vi "NI VeriStand - Close Multiple Waveforms Read Session (CDB).vi"(8 "error in (no error)":errorcluster, 11 "Multiple Waveforms Read Session (CDB)":refnum<class "Multiple Waveforms Read (CDB).lvclass">) -> (0 "error out":errorcluster)   [LabVIEW 2020, in "NI_VS Custom Device Waveform API.lvlib" / "Multiple Waveforms Read (CDB).lvclass"]
doc: "Closes a waveform read or write session. Wire data to the <B>Single Waveform Read Session (DBL)</B> input to specify the instance to use."
uses:
  Multiple Waveforms Read (CDB).lvclass
  D:/p4/penguin/lvaddon/Veristand/master/src/LabVIEW/vilib/NI VeriStand/Custom Device Waveform API/Waveform Session.lvclass
  Waveform Session.lvclass/Waveform Session.ctl
  Multiple Waveforms Read (CDB).lvclass/Multiple Waveforms Read (CDB).ctl
  Internal Comm Classes/WPL Comm/WPL Comm.lvclass/WPL Comm.ctl
  Internal Comm Classes/WPL Comm/WPL Comm (1D CDB)/WPL Comm (1D CDB).lvclass/WPL Comm (1D CDB).ctl
  Internal Comm Classes/WPL Comm/Read Access.vi
  Internal Comm Classes/WPL Comm/WPL Comm (1D CDB)/Set 1D CDB Read Q on Variant.vi
  Internal Comm Classes/WPL Comm/WPL_close waveform.vi
  Internal Comm Classes/WPL Comm/Convert Q Error to Shutdown Error.vi
  Internal Comm Classes/WPL Comm/Set ErrorQ on Variant.vi
  Internal Comm Classes/WPL Comm/Send WPL Command.vi
  Internal Comm Classes/WPL Comm/WPL Comm (1D CDB)/WPL Comm (1D CDB).lvclass
  D:/p4/penguin/lvaddon/Veristand/master/src/LabVIEW/vilib/NI VeriStand/Custom Device Waveform API/Internal Comm Classes/WPL Comm/WPL Comm.lvclass
  <vilib>/Utility/error.llb/Error Cluster From Error Code.vi
  Waveform Session.lvclass
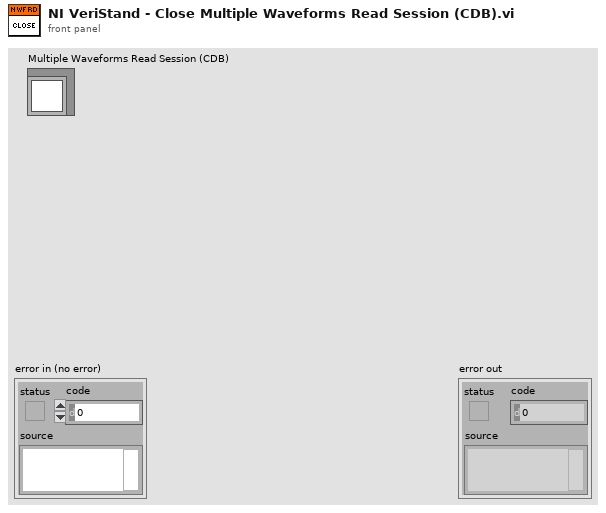
[diagram p1: front panel]
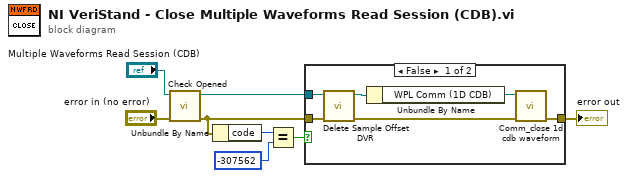
[diagram p0: block diagram]
diagram:
  n1 = call "Check Opened.vi"("error in (no error)"="error in (no error)", "Waveform Session in"="Multiple Waveforms Read Session (CDB)") -> ("error out"=w2:errorcluster, "Waveform Session out"=w6:refnum<class "Multiple Waveforms Read (CDB).lvclass">)  [unwired: 8 in]
  n2 = Unbundle By Name(w2) -> ("code"=w3:i32)
  n3 = Equal?(x=w3, y=-307562 ("error code (0)")) -> (x = y?=w1:bool)
  n4 = case shown="False" w1 {
    tunnel: w2 -> [w14 w15]
    tunnel: w6 -> [w13 _]
    tunnel: [w9 w15] -> w5
    frame False {
      n5 = call "Delete Sample Offset DVR.vi"("error in (no error)"=w14, "Waveform Session in"=w13) -> ("error out"=w10:errorcluster, "Waveform Session out"=w12:refnum<class "Multiple Waveforms Read (CDB).lvclass">)  [unwired: 8 in]
      n6 = Unbundle By Name(w12) -> ("WPL Comm (1D CDB)"=w11:refnum<class "WPL Comm (1D CDB).lvclass">)
      n7 = call "Comm_close 1d cdb waveform.vi"("error in (no error)"=w10, "WPL Comm (1D CDB) in"=w11) -> ("error out"=w9:errorcluster)  [unwired: 9 in]
    }
    frame True {
    }
  }
  "error out" <- w5
